vi "retinotopic_map_display_only_120520_svadded_fr.vi"() -> ()   [LabVIEW 2019]
uses:
  <vilib>/Utility/file.llb/Write Delimited Spreadsheet (DBL).vi
panel:
  out "WaitToStop":bool
  in  "Stop":bool
  out "Output":dbl[][](array[numeric])
  out "Display":bool=TRUE
  out "Trial":u32=1
  out "Stimuli Loaded?":bool
  out "Horizontal":bool
  out "stim_id":dbl[](array[numeric])
  out "Vertical":bool
  out "stim_loaded":dbl
  out "Elapsed Time":dbl
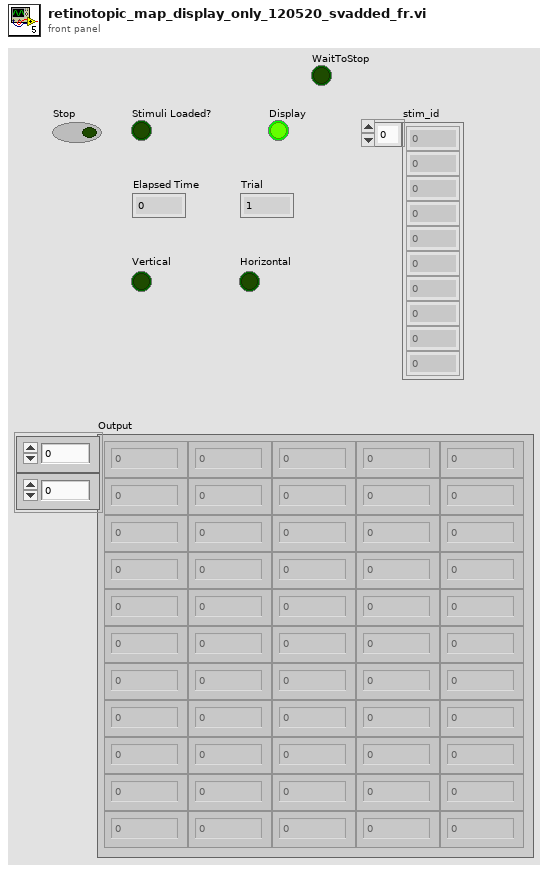
[diagram p1: front panel]
types:
  T1 = typedef "NI_Matrix.lvlib/RealMatrix.ctl" = dbl[][]
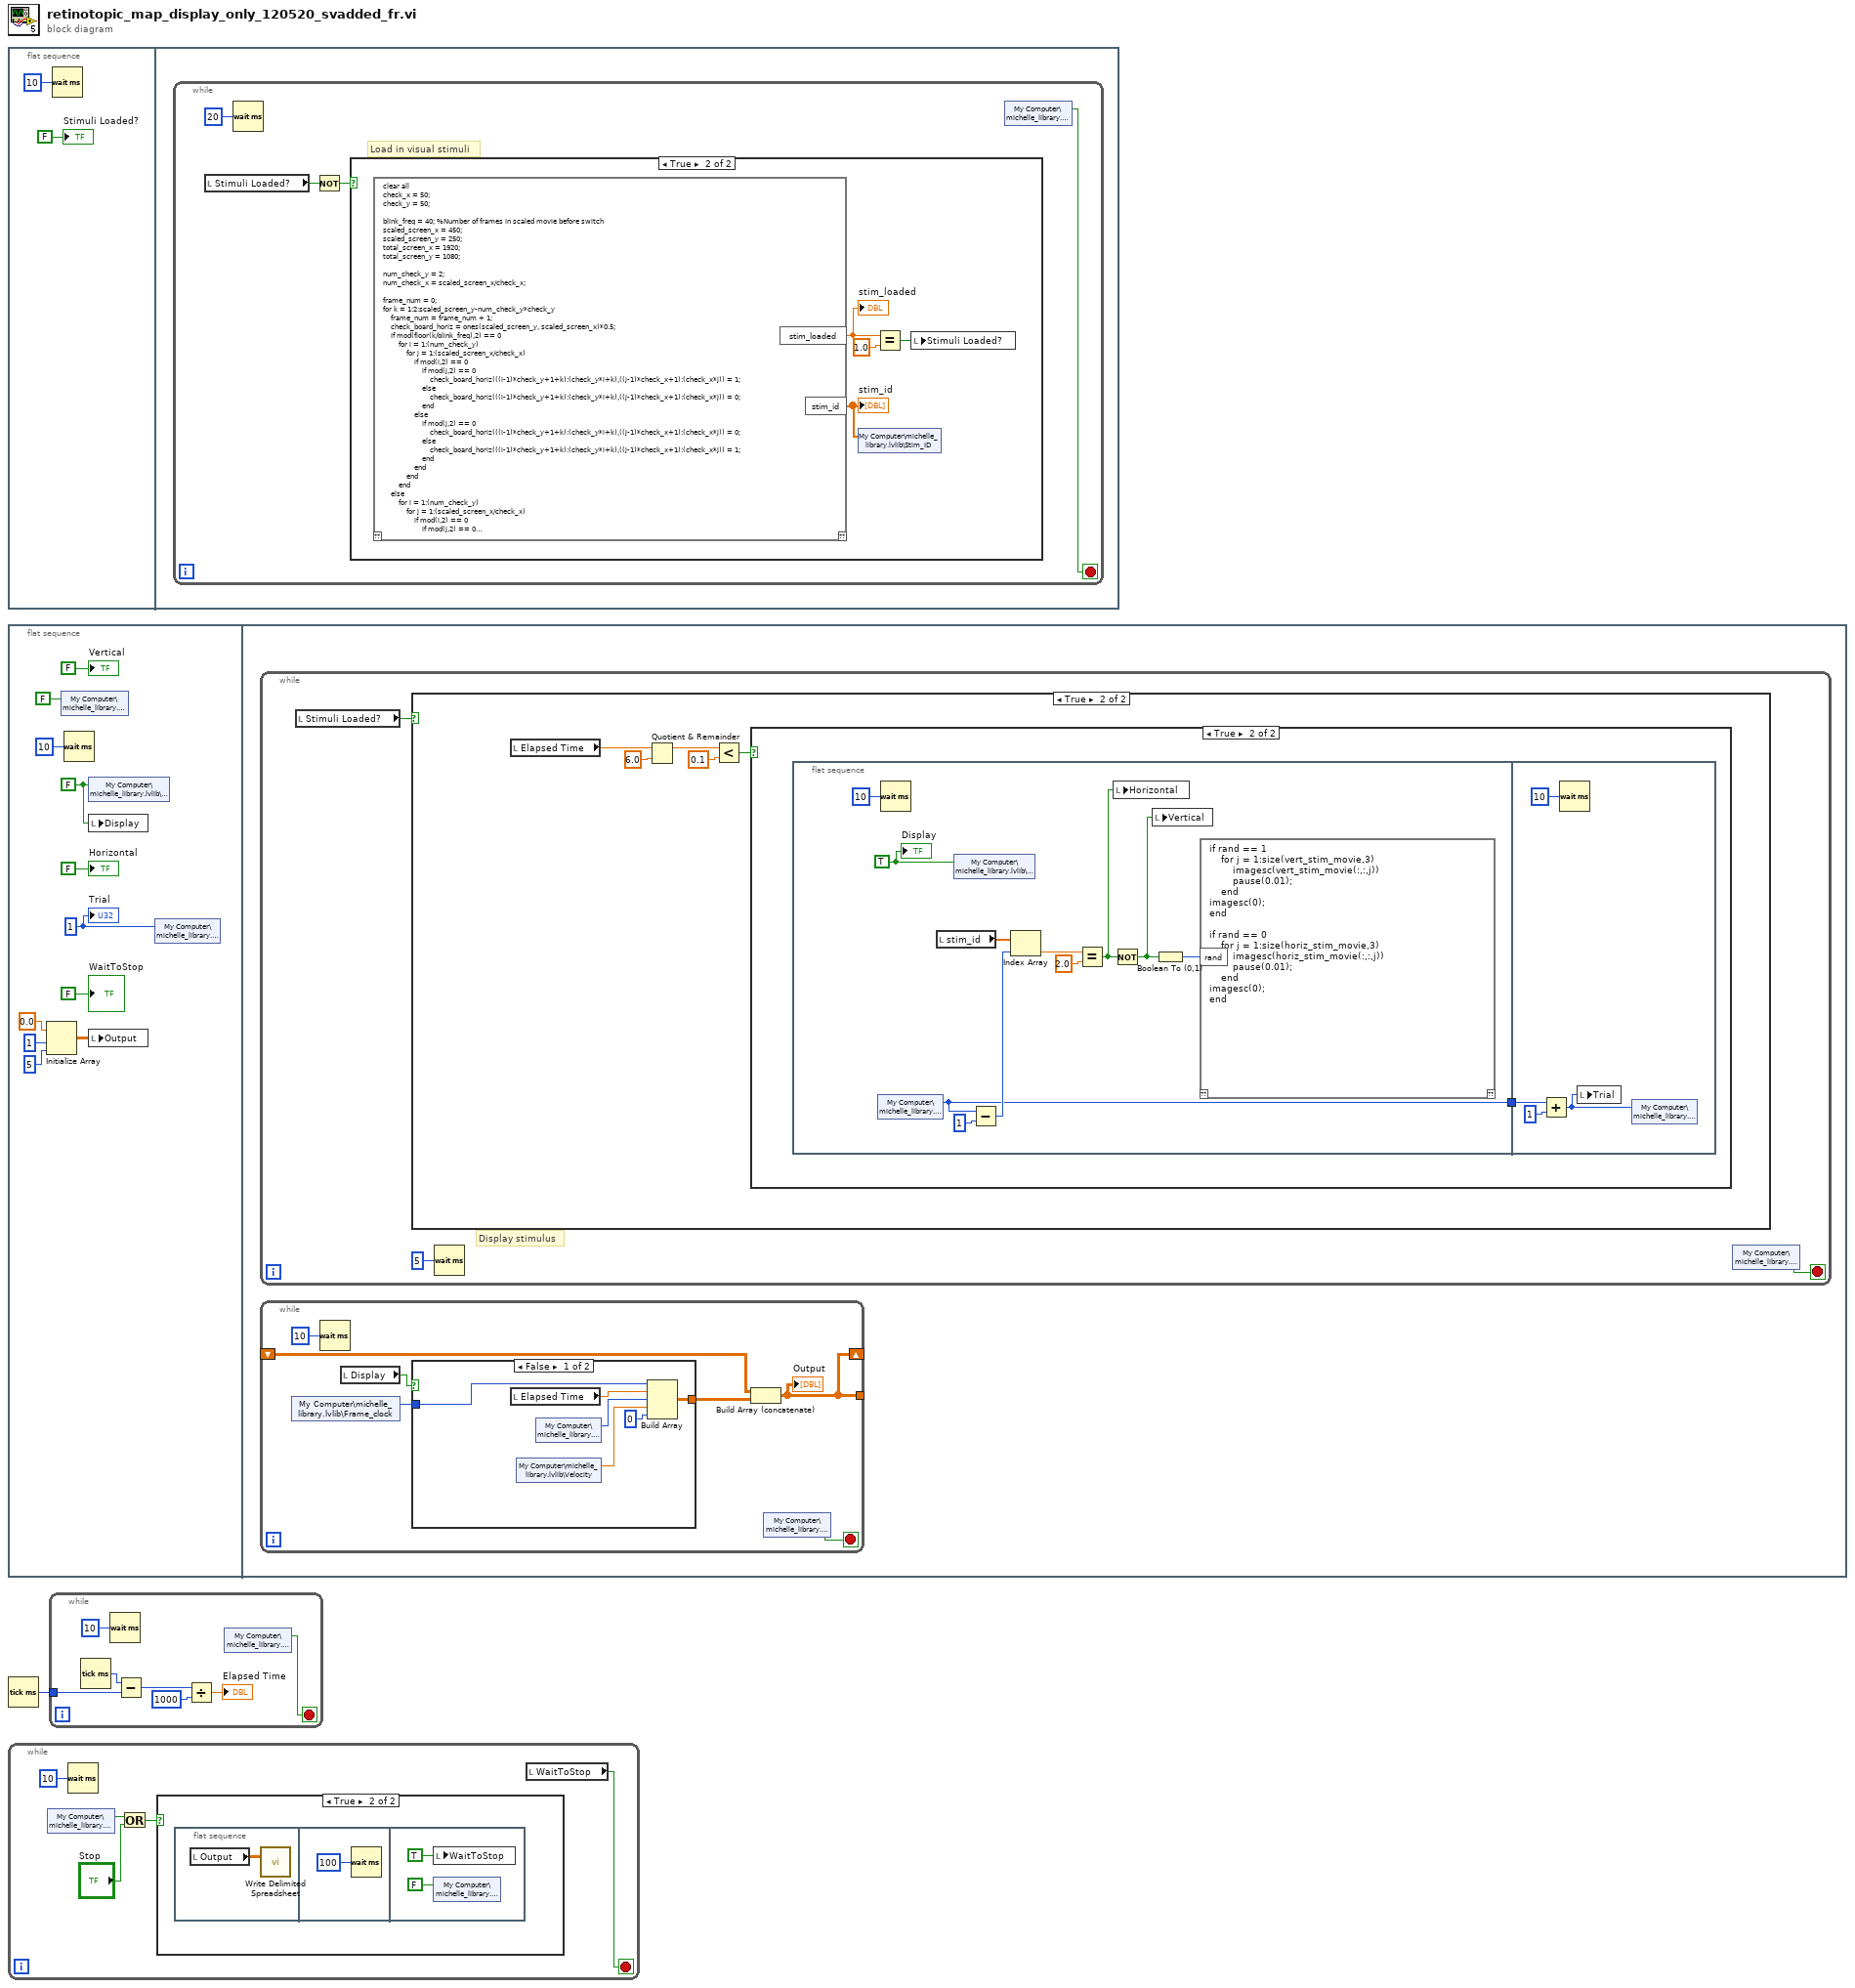
[diagram p0: block diagram]
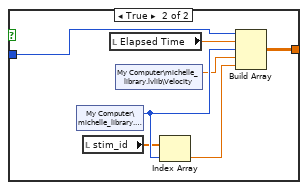
[diagram p4: hidden frame]
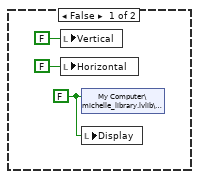
[diagram p6: hidden frame]
diagram:
  n1 = flat-sequence {
    frame #0 {
      n2 = Wait (ms)(milliseconds to wait=u32 10) -> ()  [unwired: 1 out]
      "Stimuli Loaded?" <- FALSE ("Stimuli Loaded?")
    }
    frame #1 {
      n3 = while {
        stop <- w5 stop-if-true
        # "Load in visual stimuli"
        n4 = local read "Stimuli Loaded?"() -> (w4:bool)
        n5 = Wait (ms)(milliseconds to wait=u32 20) -> ()  [unwired: 1 out]
        n6 = Not(x=w4) -> (.not. x?=w7:bool)
        n7 = case shown="True" w7 {
          frame False {
          }
          frame True {
            n8 = script code="clear all\ncheck_x = 50;\ncheck_y = 50;\n\nblink_freq = 40; %Number of frames in scaled movie before switch\nscaled_screen_x = 450;\nscaled_screen_y = 250;\ntotal_screen_x = 1920;\ntotal_screen_y = 1080;\n\nnum_check_y = 2;\nnum_check_x = scaled_screen_x/check_x;\n\nframe_num = 0;\nfor k = 1:2:scaled_screen_y-num_check_y*check_y\n    frame_num = frame_num + 1;\n    check_board_horiz = ones(scaled_screen_y, scaled_screen_x)*0.5;\n    if mod(floor(k/blink_freq),2) == 0\n        for i = 1:(num_check_y)\n            for j = 1:(scaled_screen_x/check_x)\n                if mod(i,2) == 0\n                    if mod(j,2) == 0\n                        check_board_horiz(((i-1)*check_y+1+k):(check_y*i+k),((j-1)*check_x+1):(check_x*j)) = 1;\n                    else\n                        check_board_horiz(((i-1)*check_y+1+k):(check_y*i+k),((j-1)*check_x+1):(check_x*j)) = 0;\n                    end\n                else\n                    if mod(j,2) == 0\n                        check_board_horiz(((i-1)*check_y+1+k):(check_y*i+k),((j-1)*check_x+1):(check_x*j)) = 0;\n                    else\n                        check_board_horiz(((i-1)*check_y+1+k):(check_y*i+k),((j-1)*check_x+1):(check_x*j)) = 1;\n                    end\n                end\n            end\n        end\n    else\n        for i = 1:(num_check_y)\n            for j = 1:(scaled_screen_x/check_x)\n                if mod(i,2) == 0\n                    if mod(j,2) == 0\n                        check_board_horiz(((i-1)*check_y+1+k):(check_y*i+k),((j-1)*check_x+1):(check_x*j)) = 0;\n                    else\n                        check_board_horiz(((i-1)*check_y+1+k):(check_y*i+k),((j-1)*check_x+1):(check_x*j)) = 1;\n                    end\n                else\n                    if mod(j,2) == 0\n                        check_board_horiz(((i-1)*check_y+1+k):(check_y*i+k),((j-1)*check_x+1):(check_x*j)) = 1;\n                    else\n                        check_board_horiz(((i-1)*check_y+1+k):(check_y*i+k),((j-1)*check_x+1):(check_x*j)) = 0;\n                    end\n                end\n            end\n        end\n    end\n    horiz_stim_movie(:,:,frame_num) = check_board_horiz;\nend\n\nnum_check_y = scaled_screen_y/check_y;\nnum_check_x = 2;\n\nframe_num = 0;\nfor k = 1:2:scaled_screen_x-num_check_x*check_x\n    frame_num = frame_num + 1;\n    check_board_vert = ones(scaled_screen_y, scaled_screen_x)*0.5;\n    if mod(floor(k/blink_freq),2) == 0\n        for i = 1:(num_check_x)\n            for j = 1:(scaled_screen_y/check_y)\n                if mod(i,2) == 0\n                    if mod(j,2) == 0\n                        check_board_vert(((j-1)*check_y+1):check_y*j,((i-1)*check_x+1+k):(check_x*i+k)) = 1;\n                    else\n                        check_board_vert(((j-1)*check_y+1):check_y*j,((i-1)*check_x+1+k):(check_x*i+k)) = 0;\n                    end\n                else\n                    if mod(j,2) == 0\n                        check_board_vert(((j-1)*check_y+1):check_y*j,((i-1)*check_x+1+k):(check_x*i+k)) = 0;\n                    else\n                        check_board_vert(((j-1)*check_y+1):check_y*j,((i-1)*check_x+1+k):(check_x*i+k)) = 1;\n                    end\n                end\n            end\n        end\n    else\n        for i = 1:(num_check_x)\n            for j = 1:(scaled_screen_y/check_y)\n                if mod(i,2) == 0\n                    if mod(j,2) == 0\n                        check_board_vert(((j-1)*check_y+1):check_y*j,((i-1)*check_x+1+k):(check_x*i+k)) = 0;\n                    else\n                        check_board_vert(((j-1)*check_y+1):check_y*j,((i-1)*check_x+1+k):(check_x*i+k)) = 1;\n                    end\n                else\n                    if mod(j,2) == 0\n                        check_board_vert(((j-1)*check_y+1):check_y*j,((i-1)*check_x+1+k):(check_x*i+k)) = 1;\n                    else\n                        check_board_vert(((j-1)*check_y+1):check_y*j,((i-1)*check_x+1+k):(check_x*i+k)) = 0;\n                    end\n                end\n            end\n        end\n    end\n    vert_stim_movie(:,:,frame_num) = check_board_vert;\nend\n\nset(0, 'DefaultFigurePosition', [1914 0 1940 2000]);\ncolormap(gray(256))\nset(gcf,'MenuBar','none')\nset(gca,'DataAspectRatioMode','auto')\nset(gca,'Position',[0 0 1 1])\nset(gca, 'xlimmode','manual',...\n           'ylimmode','manual',...\n           'zlimmode','manual',...\n           'climmode','manual',...\n           'alimmode','manual');\nimshow(zeros(total_screen_y,total_screen_x))\n\nstim_id = [ones(1,210)];\naltern = [1:105]*2;\nstim_id(altern) = 2;\nstim_loaded = 1;"() -> ("stim_loaded"=w11:dbl, "stim_id"=w9:dbl[])  [unwired: 1 in, 1 out]
            "stim_loaded" <- w11
            "stim_id" <- w9
            n9 = shared-variable "My Computer\\michelle_library.lvlib\\Stim_ID"(w9) -> ()  [unwired: 1 in, 1 out]
            n10 = Equal?(x=w11, y=1.0) -> (x = y?=w8:bool)
            n11 = local write "Stimuli Loaded?"(w8) -> ()
          }
        }
        n12 = shared-variable "My Computer\\michelle_library.lvlib\\Stop"() -> (w5:bool)  [unwired: 1 in, 1 out]
      }
    }
  }
  n13 = flat-sequence {
    frame #0 {
      w18 = FALSE ("Display")
      w22 = u32 1 ("Trial")
      n14 = Initialize Array(0.0 ("element"), 1 ("dimension size"), 5 ("dimension size")) -> (w14:dbl[][])
      n15 = shared-variable "My Computer\\michelle_library.lvlib\\Stop"(FALSE ("Stop")) -> ()  [unwired: 1 in, 1 out]
      n16 = Wait (ms)(milliseconds to wait=u32 10) -> ()  [unwired: 1 out]
      n17 = shared-variable "My Computer\\michelle_library.lvlib\\Display"(w18) -> ()  [unwired: 1 in, 1 out]
      n18 = local write "Display"(w18) -> ()
      n19 = local write "Output"(w14) -> ()
      n20 = shared-variable "My Computer\\michelle_library.lvlib\\Trial"(w22) -> ()  [unwired: 1 in, 1 out]
      "Horizontal" <- FALSE ("Stimulus 2")
      "Vertical" <- FALSE ("Stimulus 1")
      "Trial" <- w22
      "WaitToStop" <- FALSE
    }
    frame #1 {
      n21 = while {
        stop <- w44 stop-if-true
        # "Display stimulus"
        n22 = local read "Stimuli Loaded?"() -> (w43:bool)
        n23 = case shown="True" w43 {
          frame False {
          }
          frame True {
            n24 = local read "Elapsed Time"() -> (w50:dbl)
            n25 = Quotient & Remainder(x=w50, y=6.0) -> (x-y*floor(x/y)=w48:dbl)  [unwired: 1 out]
            n26 = Less?(x=w48, y=0.1) -> (x < y?=w46:bool)
            n27 = case shown="True" w46 {
              frame False {
                w51 = FALSE ("Display")
                n28 = local write "Vertical"(FALSE) -> ()
                n29 = local write "Horizontal"(FALSE ("Horizontal")) -> ()
                n30 = shared-variable "My Computer\\michelle_library.lvlib\\Display"(w51) -> ()  [unwired: 1 in, 1 out]
                n31 = local write "Display"(w51) -> ()
              }
              frame True {
                n32 = flat-sequence {
                  tunnel: [w56] -> w54
                  tunnel: w54 -> [w69]
                  frame #0 {
                    w60 = TRUE ("Boolean")
                    n33 = shared-variable "My Computer\\michelle_library.lvlib\\Trial"() -> (w56:u32)  [unwired: 1 in, 1 out]
                    n34 = Wait (ms)(milliseconds to wait=u32 10) -> ()  [unwired: 1 out]
                    n35 = local read "stim_id"() -> (w64:dbl[])
                    n36 = shared-variable "My Computer\\michelle_library.lvlib\\Display"(w60) -> ()  [unwired: 1 in, 1 out]
                    n37 = Subtract(x=w56, y=u32 1) -> (x-y=w57:u32)
                    n38 = Index Array(array=w64, index=w57) -> (element=w63:dbl)
                    n39 = Equal?(x=w63, y=2.0) -> (x = y?=w61:bool)
                    n40 = Not(x=w61) -> (.not. x?=w58:bool)
                    n41 = local write "Horizontal"(w61) -> ()
                    n42 = local write "Vertical"(w58) -> ()
                    n43 = Boolean To (0,1)(Boolean=w58) -> (0, 1=w59:i16)
                    n44 = script code="if rand == 1\n    for j = 1:size(vert_stim_movie,3)\n        imagesc(vert_stim_movie(:,:,j))\n        pause(0.01);\n    end\nimagesc(0);\nend\n\nif rand == 0\n    for j = 1:size(horiz_stim_movie,3)\n        imagesc(horiz_stim_movie(:,:,j))\n        pause(0.01);\n    end\nimagesc(0);\nend"("rand"=w59) -> ()  [unwired: 1 in, 1 out]
                    "Display" <- w60
                  }
                  frame #1 {
                    n45 = Add(x=w69, y=u32 1) -> (x+y=w67:u32)
                    n46 = Wait (ms)(milliseconds to wait=u32 10) -> ()  [unwired: 1 out]
                    n47 = local write "Trial"(w67) -> ()
                    n48 = shared-variable "My Computer\\michelle_library.lvlib\\Trial"(w67) -> ()  [unwired: 1 in, 1 out]
                  }
                }
              }
            }
          }
        }
        n49 = Wait (ms)(milliseconds to wait=u32 5) -> ()  [unwired: 1 out]
        n50 = shared-variable "My Computer\\michelle_library.lvlib\\Stop"() -> (w44:bool)  [unwired: 1 in, 1 out]
      }
      n51 = while {
        shift-right: [w23] -> _
        shift-left: _ -> [w26]
        tunnel: [w23] -> _
        stop <- w28 stop-if-true
        n52 = shared-variable "My Computer\\michelle_library.lvlib\\Frame_clock"() -> (w24:u32)  [unwired: 1 in, 1 out]
        n53 = Wait (ms)(milliseconds to wait=u32 10) -> ()  [unwired: 1 out]
        n54 = local read "Display"() -> (w25:bool)
        n55 = case shown="False" w25 {
          tunnel: w24 -> [w31 w42]
          tunnel: [w34 w41] -> w27
          frame False {
            n56 = local read "Elapsed Time"() -> (w33:dbl)
            n57 = shared-variable "My Computer\\michelle_library.lvlib\\Velocity"() -> (w30:dbl)  [unwired: 1 in, 1 out]
            n58 = shared-variable "My Computer\\michelle_library.lvlib\\Trial"() -> (w32:u32)  [unwired: 1 in, 1 out]
            n59 = Build Array(w31, w33, w32, w30, 0) -> (w34:T1)
          }
          frame True {
            n60 = shared-variable "My Computer\\michelle_library.lvlib\\Trial"() -> (w39:u32)  [unwired: 1 in, 1 out]
            n61 = local read "stim_id"() -> (w36:dbl[])
            n62 = local read "Elapsed Time"() -> (w40:dbl)
            n63 = shared-variable "My Computer\\michelle_library.lvlib\\Velocity"() -> (w37:dbl)  [unwired: 1 in, 1 out]
            n64 = Index Array(array=w36, index=w39) -> (element=w38:dbl)
            n65 = Build Array(w42, w40, w39, w37, w38) -> (w41:T1)
          }
        }
        n66 = Build Array (concatenate)(w26, w27) -> (w23:T1)
        "Output" <- w23
        n67 = shared-variable "My Computer\\michelle_library.lvlib\\Stop"() -> (w28:bool)  [unwired: 1 in, 1 out]
      }
    }
  }
  n68 = Tick Count (ms)() -> (millisecond timer value=w1:u32)
  n69 = while {
    stop <- w73 stop-if-true
    n70 = shared-variable "My Computer\\michelle_library.lvlib\\Stop"() -> (w71:bool)  [unwired: 1 in, 1 out]
    n71 = Wait (ms)(milliseconds to wait=u32 10) -> ()  [unwired: 1 out]
    n72 = Or(x=w71, y="Stop") -> (x .or. y?=w70:bool)
    n73 = case shown="True" w70 {
      frame False {
      }
      frame True {
        n74 = flat-sequence {
          frame #0 {
            n75 = local read "Output"() -> (w75:dbl[][])
            n76 = call-poly <vilib>:"Write Delimited Spreadsheet.vi"("2D data"=w75) -> ()  [unwired: 13 in, 2 out]
          }
          frame #1 {
            n77 = Wait (ms)(milliseconds to wait=100) -> ()  [unwired: 1 out]
          }
          frame #2 {
            n78 = local write "WaitToStop"(TRUE) -> ()
            n79 = shared-variable "My Computer\\michelle_library.lvlib\\Stop"(FALSE) -> ()  [unwired: 1 in, 1 out]
          }
        }
      }
    }
    n80 = local read "WaitToStop"() -> (w73:bool)
  }
  n81 = while {
    tunnel: w1 -> [w82]
    stop <- w79 stop-if-true
    n82 = Tick Count (ms)() -> (millisecond timer value=w83:u32)
    n83 = Wait (ms)(milliseconds to wait=u32 10) -> ()  [unwired: 1 out]
    n84 = Subtract(x=w83, y=w82) -> (x-y=w80:u32)
    n85 = Divide(x=w80, y=u32 1000) -> (x/y=→"Elapsed Time":dbl)
    n86 = shared-variable "My Computer\\michelle_library.lvlib\\Stop"() -> (w79:bool)  [unwired: 1 in, 1 out]
  }
